vi "Request Ownership.vi"(8 "error in (no error)":errorcluster, 9 "Shared Resource":bool, 10 "Dependency":refnum<class "SMO.lvclass">, 11 "SMO in":refnum<class "SMO.lvclass">) -> (0 "error out":errorcluster, 2 "Dependency out":refnum<class "SMO.lvclass">, 3 "SMO out":refnum<class "SMO.lvclass">)   [LabVIEW 2019, in "SMO.lvclass"]
doc: "JKI State Machine Objects (SMO) 1.3.0.56\nJKI - JKI\nCopyright (c) 2017, JKI"
uses:
  SMO.lvclass
  Support/Attribute.Owner/Attribute.Owner.lvclass/Attribute.Owner.ctl
  Support/Attribute.Owner/Attribute.Owner.lvclass
  C:/Users/Patrick/Documents/GitHub/Test (LV2019)/lv-venv/lv.lib/vi.lib/JKI/JKI SMO/Support/Attribute/Attribute.lvclass
  Support/Attribute.SharedResource/Attribute.SharedResource.lvclass
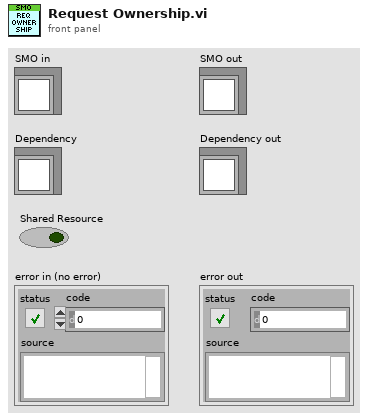
[diagram p1: front panel]
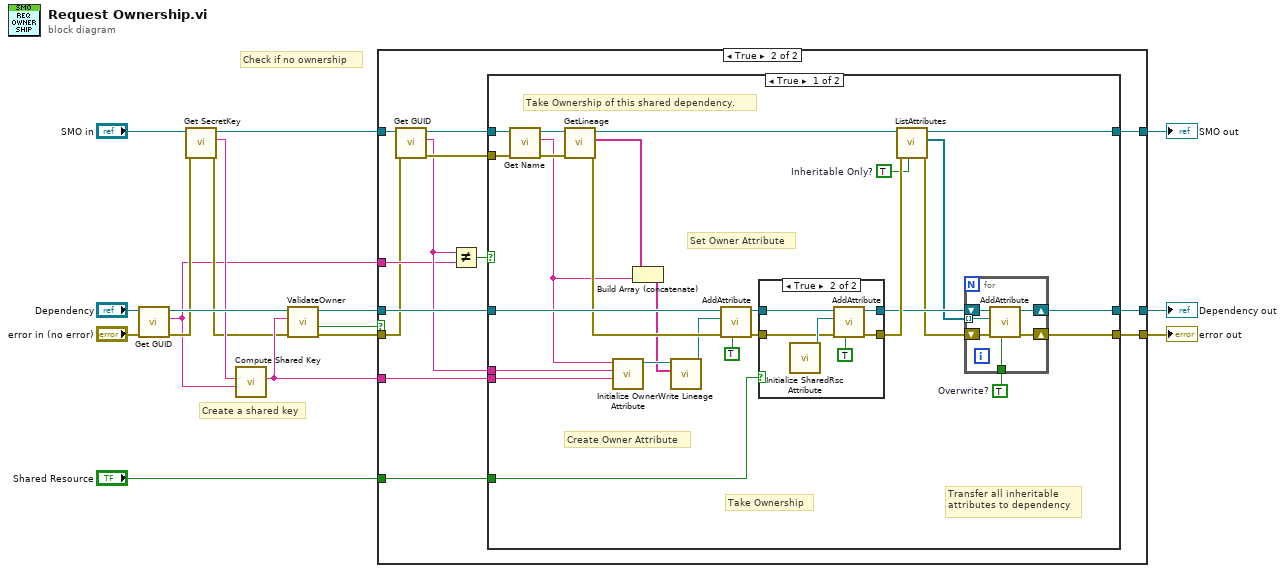
[diagram p0: block diagram]
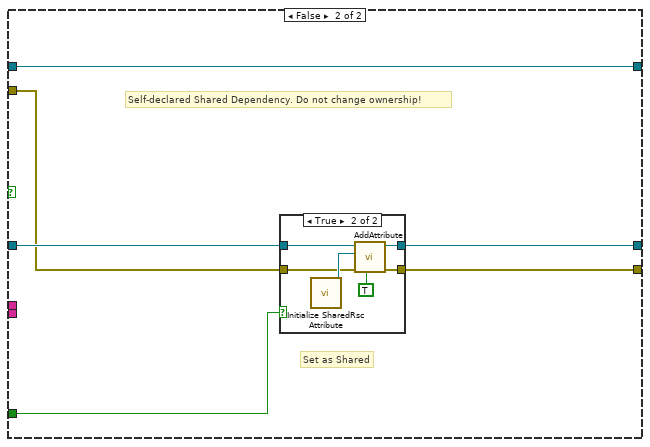
[diagram p4: hidden frame]
diagram:
  # "Check if no ownership"
  # "Create a shared key"
  n1 = call "Get GUID.vi"("error in (no error)"="error in (no error)", "SMO"="Dependency") -> ("error out"=w6:errorcluster, "GUID"=w1:string, "SMO out"=w13:refnum<class "SMO.lvclass">)  [unwired: 7 in]
  n2 = call "Get SecretKey.vi"("error in (no error)"=w6, "SMO"="SMO in") -> ("error out"=w3:errorcluster, "SecretKey"=w5:string, "SMO out"=w4:refnum<class "SMO.lvclass">)  [unwired: 7 in]
  n3 = call "Compute Shared Key.vi"("GUID"=w1, "SecretKey"=w5) -> ("Shared Key"=w15:string)  [unwired: 9 in]
  n4 = call "ValidateOwner.vi"("error in (no error)"=w3, "Shared Key"=w15, "SMO in"=w13) -> ("error out"=w16:errorcluster, "not set"=w2:bool, "SMO out"=w14:refnum<class "SMO.lvclass">)  [unwired: 5 in, 1 out]
  n5 = case shown="True" w2 {
    tunnel: [w20 w30] -> w17
    tunnel: w4 -> [w20 w27]
    tunnel: "Shared Resource" -> [_ w33]
    tunnel: [w19 w29] -> w11
    tunnel: [w18 w28] -> w12
    tunnel: w14 -> [w19 w32]
    tunnel: w15 -> [_ w31]
    tunnel: w16 -> [w18 w21]
    tunnel: w1 -> [_ w23]
    frame False {
      # "Already Owned by other SMO"
    }
    frame True {
      n6 = call "Get GUID.vi"("error in (no error)"=w21, "SMO"=w27) -> ("error out"=w25:errorcluster, "GUID"=w24:string, "SMO out"=w26:refnum<class "SMO.lvclass">)  [unwired: 7 in]
      n7 = Not Equal?(x=w24, y=w23) -> (x != y?=w22:bool)
      n8 = case shown="True" w22 {
        tunnel: w33 -> [w60 w80]
        tunnel: w32 -> [w57 w79]
        tunnel: w31 -> [w56 _]
        tunnel: [w55 w77] -> w30
        tunnel: [w52 w76] -> w29
        tunnel: [w49 w75] -> w28
        tunnel: w26 -> [w36 w77]
        tunnel: w25 -> [w35 w78]
        tunnel: w24 -> [w34 _]
        frame True {
          w48 = TRUE  # Overwrite?
          w53 = TRUE  # Inheritable Only?
          # "Take Ownership of this shared dependency."
          # "Transfer all inheritable\nattributes to dependency"
          # "Take Ownership"
          # "Create Owner Attribute"
          # "Set Owner Attribute"
          n9 = call "Get Name.vi"("error in (no error)"=w35, "SMO"=w36) -> ("error out"=w43:errorcluster, "Name"=w38:string, "SMO out"=w45:refnum<class "SMO.lvclass">)  [unwired: 7 in]
          n10 = call "GetLineage.vi"("error in (no error)"=w43, "SMO in"=w45) -> ("error out"=w42:errorcluster, "Lineage"=w39:string[], "SMO out"=w44:refnum<class "SMO.lvclass">)  [unwired: 7 in]
          n11 = call "Initialize Owner Attribute.vi"("Shared Key"=w56, "Owner GUID"=w34, "Owner Name"=w38) -> ("Attribute.Owner"=w41:refnum<class "Attribute.Owner.lvclass">)  [unwired: 8 in]
          n12 = Build Array (concatenate)(w39, w38) -> (w37:string[])
          n13 = call "Write Lineage.vi"("Lineage"=w37, "Attribute.Owner in"=w41) -> ("Attribute.Owner out"=w40:refnum<class "Attribute.Owner.lvclass">)  [unwired: 8 in, 1 out]
          n14 = call "AddAttribute.vi"("Overwrite? (F)"=TRUE, "error in (no error)"=w42, "Attribute"=w40, "SMO in"=w57) -> ("error out"=w59:errorcluster, "SMO out"=w58:refnum<class "SMO.lvclass">)  [unwired: 6 in]
          n15 = case shown="True" w60 {
            tunnel: w58 -> [w68 w74]
            tunnel: [w68 w73] -> w51
            tunnel: w59 -> [w67 w71]
            tunnel: [w67 w70] -> w54
            frame False {
            }
            frame True {
              n16 = call "Initialize SharedRsc Attribute.vi"() -> ("Attribute.SharedResource"=w72:refnum<class "Attribute.SharedResource.lvclass">)  [unwired: 11 in]
              n17 = call "AddAttribute.vi"("Overwrite? (F)"=TRUE, "error in (no error)"=w71, "Attribute"=w72, "SMO in"=w74) -> ("error out"=w70:errorcluster, "SMO out"=w73:refnum<class "SMO.lvclass">)  [unwired: 6 in]
            }
          }
          n18 = call "ListAttributes.vi"("Inheritable Only? (F: all)"=w53, "error in (no error)"=w54, "SMO in"=w44) -> ("error out"=w50:errorcluster, "[Attributes]"=w47:refnum<class "Attribute.lvclass">[], "SMO out"=w55:refnum<class "SMO.lvclass">)  [unwired: 6 in]
          n19 = for {
            tunnel: w48 -> [w62]
            shift-right: [w66] -> w52
            shift-left: w51 -> [w65]
            shift-right: [w63] -> w49
            shift-left: w50 -> [w64]
            tunnel: w47 -> [w61] mode=indexing
            n20 = call "AddAttribute.vi"("Overwrite? (F)"=w62, "error in (no error)"=w64, "Attribute"=w61, "SMO in"=w65) -> ("error out"=w63:errorcluster, "SMO out"=w66:refnum<class "SMO.lvclass">)  [unwired: 6 in]
          }
        }
        frame False {
          # "Self-declared Shared Dependency. Do not change ownership!"
          # "Set as Shared"
          n21 = case shown="True" w80 {
            tunnel: w79 -> [w82 w88]
            tunnel: [w82 w87] -> w76
            tunnel: w78 -> [w81 w85]
            tunnel: [w81 w84] -> w75
            frame False {
            }
            frame True {
              n22 = call "Initialize SharedRsc Attribute.vi"() -> ("Attribute.SharedResource"=w86:refnum<class "Attribute.SharedResource.lvclass">)  [unwired: 11 in]
              n23 = call "AddAttribute.vi"("Overwrite? (F)"=TRUE, "error in (no error)"=w85, "Attribute"=w86, "SMO in"=w88) -> ("error out"=w84:errorcluster, "SMO out"=w87:refnum<class "SMO.lvclass">)  [unwired: 6 in]
            }
          }
        }
      }
    }
  }
  "SMO out" <- w17
  "error out" <- w12
  "Dependency out" <- w11
